vi "Write Analog In.vi"(8 "error in (no error)":errorcluster, 10 "Analog In":dbl[](array[numeric]), 11 "PLC in":refnum<class "PLC.lvclass">) -> (0 "error out":errorcluster, 3 "PLC out":refnum<class "PLC.lvclass">)   [LabVIEW 2018, in "PLC.lvlib" / "PLC.lvclass"]
uses:
  PLC.lvclass
  PLC.lvclass/PLC.ctl
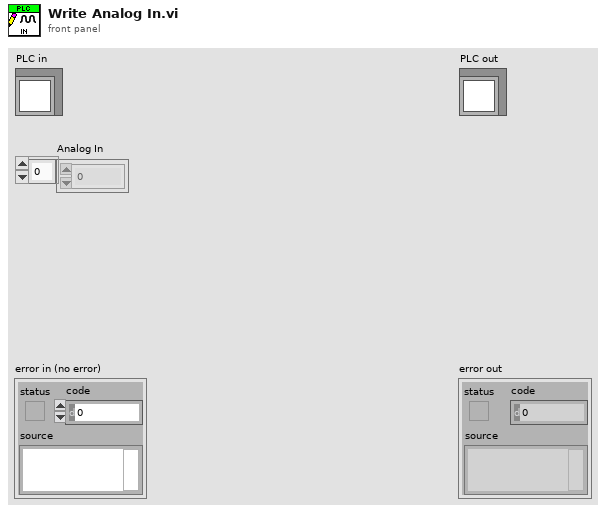
[diagram p1: front panel]
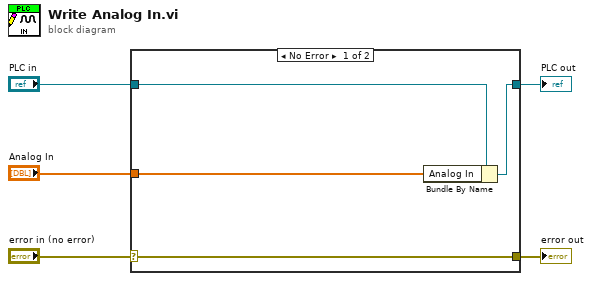
[diagram p0: block diagram]
diagram:
  n1 = case shown="No Error" "error in (no error)" {
    selector: "error in (no error)" -> [w9 w10]
    tunnel: [w9 w10] -> w4
    tunnel: [w7 w11] -> w2
    tunnel: "PLC in" -> [w8 w11]
    tunnel: "Analog In" -> [w6 _]
    frame No Error {
      n2 = Bundle By Name(cluster=w8, "Analog In"=w6) -> (w7:refnum<class "PLC.lvclass">)
    }
    frame Error {
    }
  }
  "error out" <- w4
  "PLC out" <- w2
